vi "ConnectWifiMention.vi"(5 "Slot":T1, 7 "error out":errorcluster, 9 "WIFI":string) -> (0 "错误输出":errorcluster, 2 "连接结果":bool)   [LabVIEW 2013]
uses:
  SystemCode/SysControl/Slot.ctl
panel:
  out "提示":string
  out "Wi-FI名称":string
  in  "PASS":bool
  in  "停止":bool
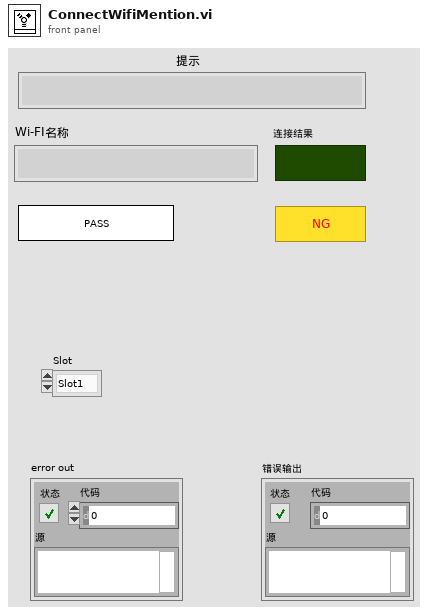
[diagram p1: front panel]
types:
  T1 = typedef "Slot.ctl" = enum16{"Slot1", "Slot2", "Slot3", "Slot4"}
  T2 = typedef "LVRectTypeDef.ctl" = cluster{"Left":i16, "Top":i16, "Right":i16, "Bottom":i16}
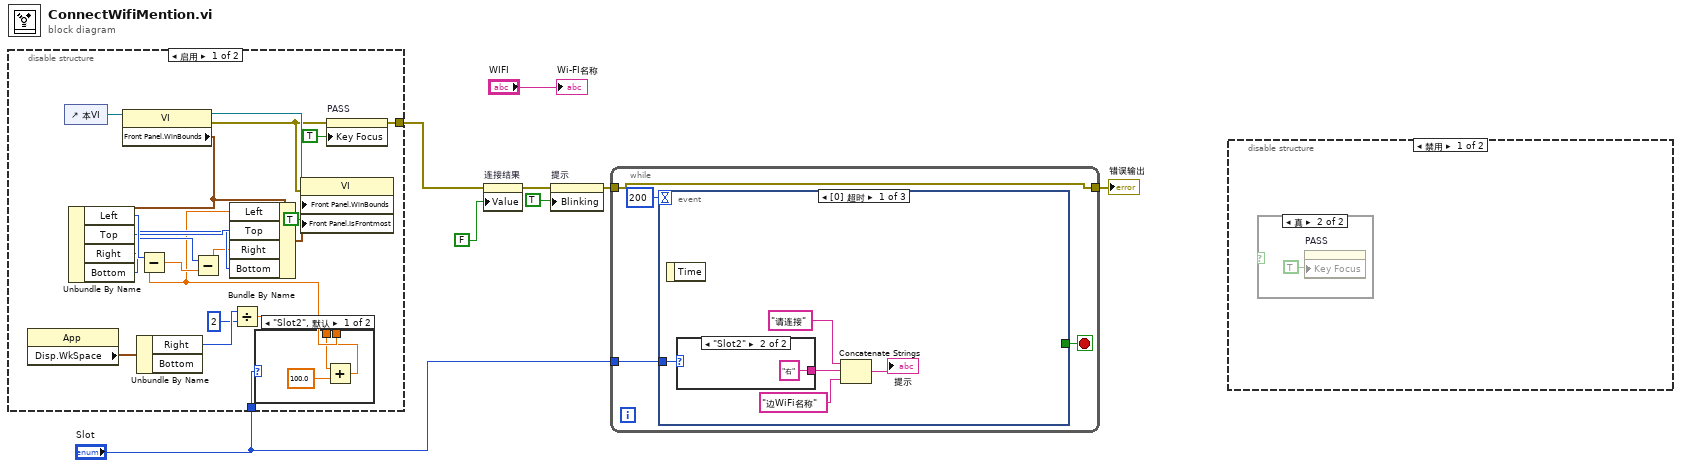
[diagram p0: block diagram]
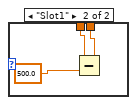
[diagram p4: hidden frame]
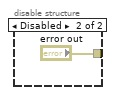
[diagram p5: hidden frame]
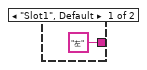
[diagram p6: hidden frame]
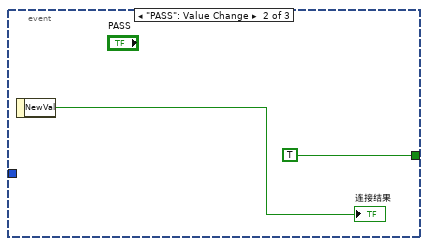
[diagram p7: hidden frame]
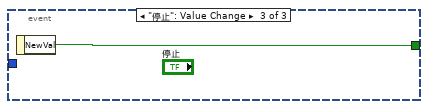
[diagram p8: hidden frame]
diagram:
  n1 = disable-structure shown="启用" {
    disable-tunnel: [w10 "error out"] -> w3
    disable-tunnel: "Slot" -> [w12 _]
    frame Enabled {
      n2 = property class="App"() -> ("Disp.WkSpace"=w25:T2)  [unwired: 2 in, 2 out]
      n3 = control-ref of="本VI"() -> (w28:refnum<vi>)
      n4 = property class="VI"(reference=w28) -> (reference out=w27:refnum<vi>, error out=w11:errorcluster, "Front Panel.WinBounds"=w23:T2)  [unwired: 1 in]
      n5 = Unbundle By Name(w23) -> ("Left"=w22:i16, "Top"=w21:i16, "Right"=w19:i16, "Bottom"=w20:i16)
      n6 = Unbundle By Name(w25) -> ("Right"=w16:i16)  [unwired: 1 out]
      n7 = Divide(x=w16, y=i16 2) -> (x/y=w14:dbl)
      n8 = case shown="\"Slot2\", 默认" w12 {
        tunnel: w14 -> [w31 w34]
        tunnel: [w29 w32] -> w13
        frame "Slot2", Default {
          n9 = Add(x=w31, y=100.0) -> (x+y=w29:dbl)
        }
        frame "Slot1" {
          n10 = Subtract(x=w34, y=500.0) -> (x-y=w32:dbl)
        }
      }
      n11 = Subtract(x=w22, y=w13) -> (x-y=w18:dbl)
      n12 = Subtract(x=w19, y=w18) -> (x-y=w17:dbl)
      n13 = Bundle By Name(cluster=w23, "Left"=w13, "Top"=w21, "Right"=w17, "Bottom"=w20) -> (w26:T2)
      n14 = property class="VI"(reference=w27, error in=w11, "Front Panel.WinBounds"=w26, "Front Panel.IsFrontmost"=TRUE ("前面板窗口:可调整大小")) -> ()  [unwired: 2 out]
      n15 = property on="PASS" class="Bool"(error in=w11, "Key Focus"=TRUE ("键选中")) -> (error out=w10:errorcluster)  [unwired: 1 in, 1 out]
    }
    frame Disabled {
    }
  }
  n16 = property on="连接结果" class="Bool (严格)"(error in=w3, "Value"=FALSE ("比对结果")) -> (error out=w5:errorcluster)  [unwired: 1 in, 1 out]
  n17 = property on="提示" class="Str"(error in=w5, "Blinking"=TRUE ("闪烁")) -> (error out=w8:errorcluster)  [unwired: 1 in, 1 out]
  n18 = while {
    tunnel: w8 -> [w37]
    tunnel: [w37] -> w4
    tunnel: "Slot" -> [w36]
    stop <- w39 stop-if-true
    n19 = event shown="[0] 超时" {
      selector: _ -> [_ _ _]
      dyn-events: _ -> [_ _ _]
      timeout: 200 -> [_ _ _]
      tunnel: [_ TRUE w49] -> w39
      tunnel: w36 -> [w40 _ _]
      event Timeout {
        n20 = event-data() -> ()  [unwired: 1 in, 1 out]
        n21 = case shown="\"Slot2\"" w40 {
          tunnel: ["左" ("字符串") "右" ("字符串")] -> w41
          frame "Slot1", Default {
          }
          frame "Slot2" {
          }
        }
        n22 = Concatenate Strings("请连接" ("字符串"), w41, "边WiFi名称" ("字符串")) -> (→"提示":string)
      }
      event "PASS": Value Change {
        n23 = event-data() -> ("NewVal"=→"连接结果":bool)  [unwired: 1 in]
      }
      event "停止": Value Change {
        n24 = event-data() -> ("NewVal"=w49:bool)  [unwired: 1 in]
      }
    }
  }
  "错误输出" <- w4
  n25 = disable-structure shown="禁用" {
    frame Disabled {
      n26 = case shown="真" {
        selector: _ -> [_ _]
        frame False {
        }
        frame True {
          n27 = property on="PASS" class="Bool"("Key Focus"=TRUE ("键选中")) -> ()  [unwired: 2 in, 2 out]
        }
      }
    }
    frame Enabled {
    }
  }
  "Wi-FI名称" <- "WIFI"
